vi "20170411-lecture3-3 flat seq.vi"() -> ()   [LabVIEW 2014]
panel:
  out "total time spent (ms)":u32
  in  "generate random number":i32
  out "Waveform Chart":dbl(graph)
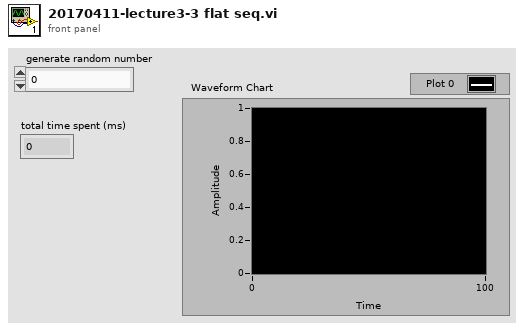
[diagram p1: front panel]
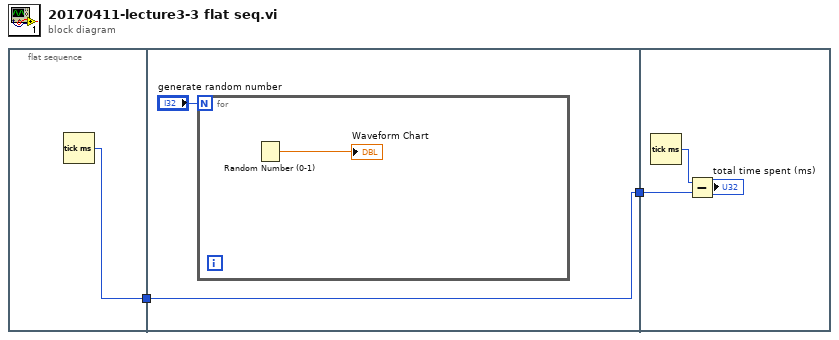
[diagram p0: block diagram]
diagram:
  n1 = flat-sequence {
    tunnel: [w3] -> w2
    tunnel: w2 -> [w4]
    tunnel: [w4] -> w1
    tunnel: w1 -> [w8]
    frame #0 {
      n2 = Tick Count (ms)() -> (millisecond timer value=w3:u32)
    }
    frame #1 {
      n3 = for {
        N: "generate random number" -> [_]
        n4 = Random Number (0-1)() -> (number: 0 to 1=→"Waveform Chart":dbl)
      }
    }
    frame #2 {
      n5 = Tick Count (ms)() -> (millisecond timer value=w9:u32)
      n6 = Subtract(x=w9, y=w8) -> (x-y=→"total time spent (ms)":u32)
    }
  }
